vi "updateSoundSettings.vi"(8 "error in (no error)":errorcluster, 10 "duration":dbl=1.0 format="%0.2f", 11 "Sound in":refnum<class "Sound.lvclass">) -> (0 "error out":errorcluster, 3 "Sound out":refnum<class "Sound.lvclass">)   [LabVIEW 2019, in "Sound.lvclass"]
uses:
  Sound.lvclass
  Sound.lvclass/Sound.ctl
  <vilib>/Waveform/WDTOps.llb/WDT Get Waveform Subset DBL.vi
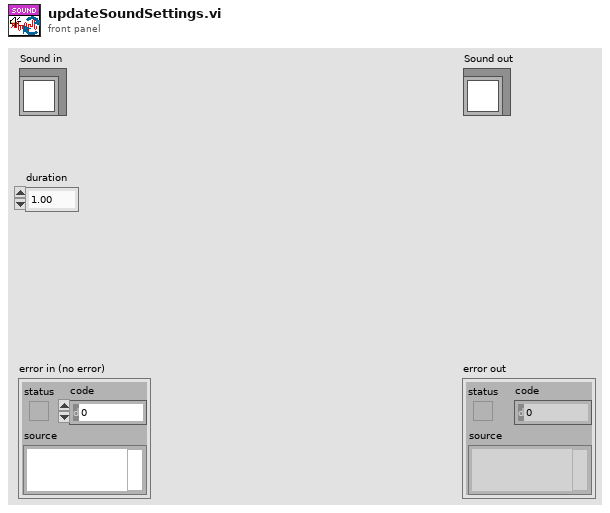
[diagram p1: front panel]
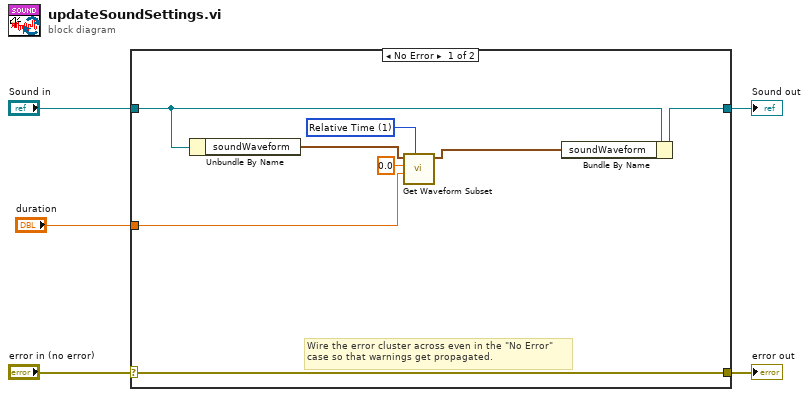
[diagram p0: block diagram]
diagram:
  n1 = case shown="No Error" "error in (no error)" {
    selector: "error in (no error)" -> [w13 w15]
    tunnel: [w13 w15] -> w4
    tunnel: [w11 w14] -> w2
    tunnel: "Sound in" -> [w12 w14]
    tunnel: "duration" -> [w7 _]
    frame No Error {
      w9 = u16 1 items=["Samples", "Relative Time"] ("start/duration format")
      # "Wire the error cluster across even in the \"No Error\"\ncase so that warnings get propagated."
      n2 = Unbundle By Name(w12) -> ("soundWaveform"=w10:waveform(dbl))
      n3 = call-poly <vilib>:"Get Waveform Subset.vi"("start/duration format"=w9, "duration"=w7, "start samples/time"=0.0, "waveform in"=w10) -> ("waveform out"=w6:waveform(dbl))  [unwired: 2 in, 3 out]
      n4 = Bundle By Name(cluster=w12, "soundWaveform"=w6) -> (w11:refnum<class "Sound.lvclass">)
    }
    frame Error {
    }
  }
  "error out" <- w4
  "Sound out" <- w2
